vi "SetCaption.vi"(8 "error in (no error)":errorcluster, 10 "Caption":string, 11 "Progress in":refnum<class "Progress.lvclass">) -> (0 "error out":errorcluster, 3 "Progress out":refnum<class "Progress.lvclass">)   [LabVIEW 2021, in "Progress.lvlib" / "Progress.lvclass"]
uses:
  Progress.lvclass
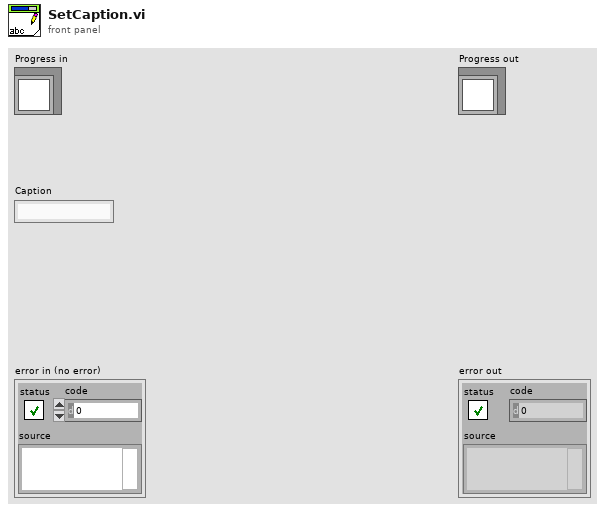
[diagram p1: front panel]
types:
  T1 = typedef "Progress.lvlib/Progress.lvclass/Data.ctl" = cluster{"SlideRefnum":refnum<vi>, "ProgressValue":u64, "NbElement":u64, "Caption":string, "UINotifier":refnum<notifier>, "StopUI":refnum<user-event>}
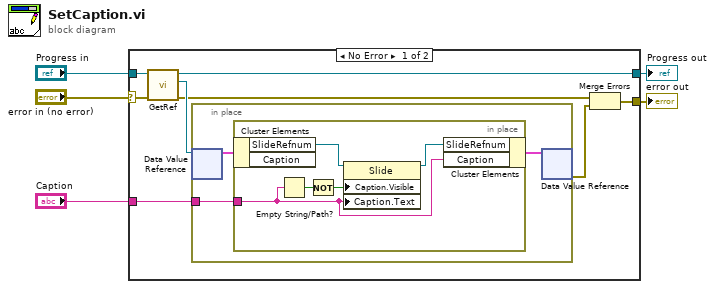
[diagram p0: block diagram]
diagram:
  n1 = case shown="No Error" "error in (no error)" {
    selector: "error in (no error)" -> [w8 w23]
    tunnel: [w7 w23] -> w4
    tunnel: [w10 w22] -> w2
    tunnel: "Progress in" -> [w9 w22]
    tunnel: "Caption" -> [w6 _]
    frame No Error {
      n2 = call "GetRef.vi"("error in (no error)"=w8, "Progress in"=w9) -> ("error out"=w11:errorcluster, "ref"=w13:refnum<data-value>, "Progress out"=w10:refnum<class "Progress.lvclass">)  [unwired: 7 in]
      n3 = in-place {
        in-place-border: w6 -> [w14]
        n4 = in-place-dvr #1(w13) -> (w16:T1)  [unwired: 1 out]
        n5 = in-place {
          in-place-border: w14 -> [w17]
          n6 = in-place-cluster #2(w16) -> ("SlideRefnum"=w21:refnum<vi>)  [unwired: 1 out]
          n7 = Empty String/Path?(string/path=w17) -> (empty?=w19:bool)
          n8 = Not(x=w19) -> (.not. x?=w18:bool)
          n9 = property class="Slide"(reference=w21, "Caption.Visible"=w18, "Caption.Text"=w17) -> (reference out=w20:refnum<vi>)  [unwired: 1 in, 1 out]
          n10 = in-place-cluster #2("SlideRefnum"=w20, "Caption"=w17) -> (w15:T1)
        }
        n11 = in-place-dvr #1(w15) -> (w12:errorcluster)  [unwired: 1 out]
      }
      n12 = Merge Errors(w11, w12) -> (w7:errorcluster)
    }
    frame Error {
    }
  }
  "error out" <- w4
  "Progress out" <- w2
